vi "Convert Launch Type from gRPC Type.vi"(11 "Loader Type":T1) -> (2 "Valid":bool, 3 "Loader Type":T2)   [LabVIEW 2021, in "CIFPluginManager.lvclass"]
uses:
  CIFPluginManager.lvclass
  CIFPluginManager.lvclass/CIFPluginManager.ctl
  typedef/Loader Type.ctl
  gRPC/CIF_Manager_server/RPC Messages/cif_management_common_LoaderType.ctl
  gRPC/CIF_Manager_server/CIF_Manager_server.lvlib
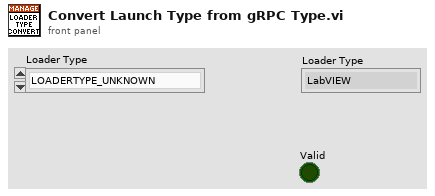
[diagram p1: front panel]
types:
  T1 = typedef "CIF_Manager_server.lvlib/cif_management_common_LoaderType.ctl" = enum32{"LOADERTYPE_UNKNOWN", "LOADERTYPE_LABVIEW"}
  T2 = typedef "CIFPluginManager.lvclass/Loader Type.ctl" = enum16{"LabVIEW"}
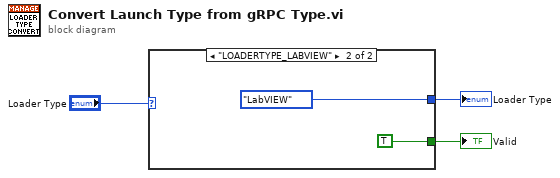
[diagram p0: block diagram]
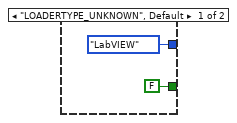
[diagram p2: hidden frame]
diagram:
  n1 = case shown="\"LOADERTYPE_LABVIEW\"" "Loader Type" {
    tunnel: [Loader_Type."LabVIEW" ("Launcher Type") Loader_Type."LabVIEW" ("Launcher Type")] -> w2
    tunnel: [FALSE TRUE] -> w1
    frame "LOADERTYPE_UNKNOWN", Default {
    }
    frame "LOADERTYPE_LABVIEW" {
    }
  }
  "Loader Type" <- w2
  "Valid" <- w1
